vi "Common-ModifyBoolCaptionTextAndColor.vi"(9 "标题.文本颜色:文本颜色数组":u32[](array[numeric]), 10 "标题.文本数组":string[](array[string]), 11 "引用数组":refnum<vi>[](array[refnum])) -> ()   [LabVIEW 2014]
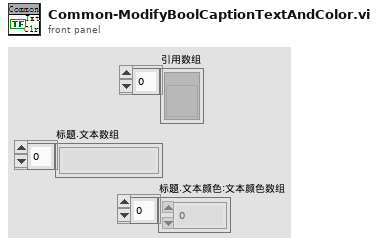
[diagram p1: front panel]
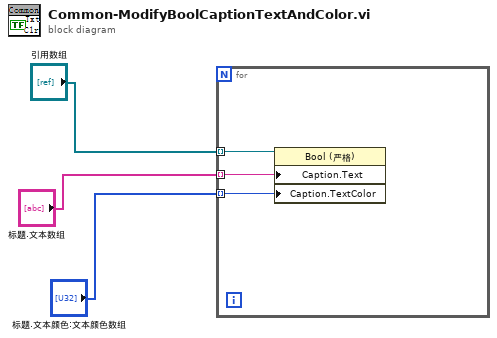
[diagram p0: block diagram]
diagram:
  n1 = for {
    tunnel: "引用数组" -> [w6] mode=indexing
    tunnel: "标题.文本数组" -> [w5] mode=indexing
    tunnel: "标题.文本颜色:文本颜色数组" -> [w4] mode=indexing
    n2 = property class="Bool (严格)"(reference=w6, "Caption.Text"=w5, "Caption.TextColor"=w4) -> ()  [unwired: 1 in, 2 out]
  }
